vi "Configure Value (IO).vi"(0 "VISA resource name":refnum<visa-resource-name>, 5 "Channel (0001)":string="0001", 7 "Display Characters Of Lower Limit (\"\")":string, 9 "Display Characters Of Upper Limit (\"\")":string, 11 "error in (no error)":errorcluster) -> (4 "VISA resource name out":refnum<visa-resource-name>, 6 "Channel":string, 15 "error out":errorcluster)   [LabVIEW 2020, in "Yokogawa GX Series.lvlib"]
doc: "Sets the upper/lower limit display characters of DI channel or DO channel.\n\nCommand: SValueIO"
uses:
  <instrlib>/Yokogawa GX Series/Yokogawa GX Series.lvlib
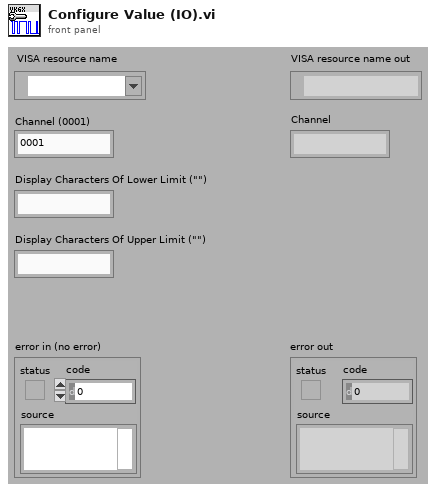
[diagram p1: front panel]
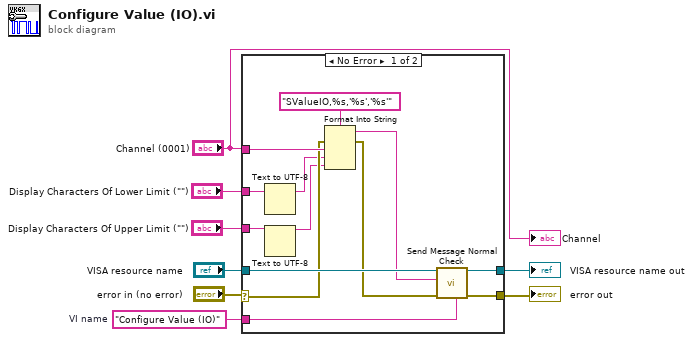
[diagram p0: block diagram]
diagram:
  w7 = "Configure Value (IO)"  # VI name
  n1 = case shown="No Error" "error in (no error)" {
    selector: "error in (no error)" -> [w13 w22]
    tunnel: "VISA resource name" -> [w21 w23]
    tunnel: w7 -> [w20 _]
    tunnel: [w19 w23] -> w6
    tunnel: [w18 w22] -> w5
    tunnel: "Display Characters Of Lower Limit (\"\")" -> [w12 _]
    tunnel: "Display Characters Of Upper Limit (\"\")" -> [w10 _]
    tunnel: "Channel (0001)" -> [w14 _]
    frame No Error {
      n2 = Text to UTF-8(11:w12) -> (3:w11:string)  [unwired: 2 in, 1 out]
      n3 = Text to UTF-8(11:w10) -> (3:w9:string)  [unwired: 2 in, 1 out]
      n4 = Format Into String(format string="SValueIO,%s,'%s','%s'", error in=w13, w14, w11, w9) -> (resulting string=w15:string, error out=w16:errorcluster)  [unwired: 1 in]
      n5 = call <instrlib>:"Send Message Normal Check.vi"("Source (\"\")"=w20, "error in (no error)"=w16, "Send Message (\"\")"=w15, "VISA resource name"=w21) -> ("error out"=w18:errorcluster, "VISA resource name out"=w19:refnum<visa-resource-name>)  [unwired: 2 in, 4 out]
    }
    frame Error {
    }
  }
  "error out" <- w5
  "VISA resource name out" <- w6
  "Channel" <- "Channel (0001)"
